vi "PS_Pressure_Cal.vi"(11 "P":dbl=1.0) -> (0 "error out":errorcluster, 3 "Pn":dbl)   [LabVIEW 2011]
uses:
  PS_Global.vi
panel:
  # "torr"
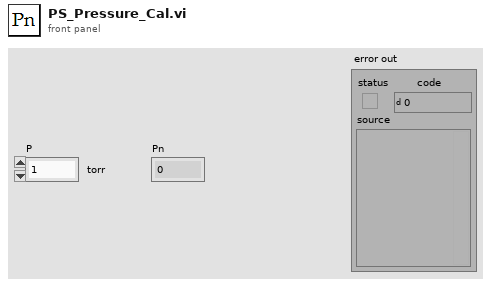
[diagram p1: front panel]
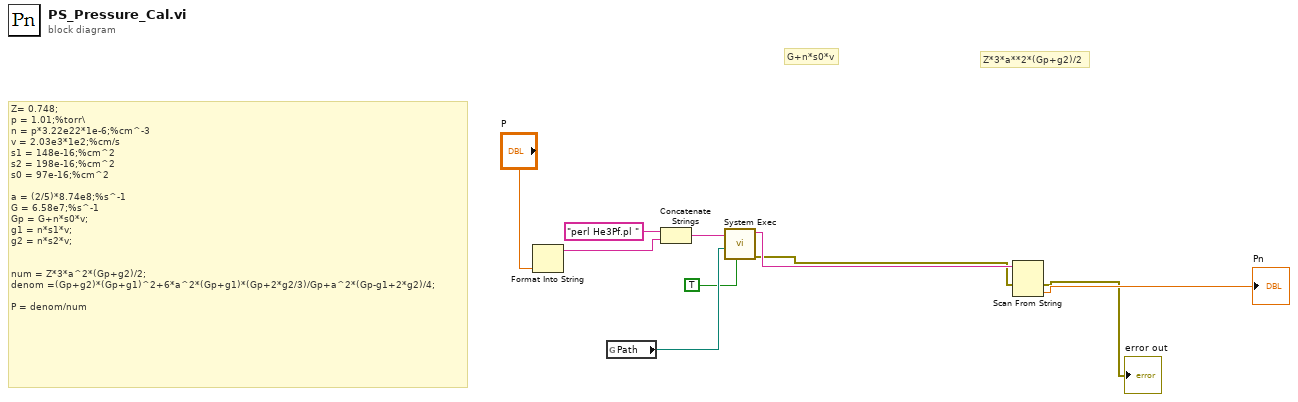
[diagram p0: block diagram]
diagram:
  # "G+n*s0*v"
  # "Z*3*a**2*(Gp+g2)/2"
  # "Z= 0.748;\np = 1.01;%torr\\\nn = p*3.22e22*1e-6;%cm^-3\nv = 2.03e3*1e2;%cm/s\ns1 = 148e-16;%cm^2\ns2 = 198e-16;%cm^2\ns0 = 97e-16;%cm^2\n\na = (2/5)*8.74e8;%s^-1\nG = 6.58e7;%s^-1\nGp = G+n*s0*v;\ng1 = n*s1*v;\ng2 = n*s2*v;\n\n\nnum = Z*3*a^2*(Gp+g2)/2;\ndenom =(Gp+g2)*(Gp+g1)^2+6*a^2*(Gp+g1)*(Gp+2*g2/3)/Gp+a^2*(Gp-g1+2*g2)/4;\n\nP = denom/num"
  n1 = Format Into String("P") -> (resulting string=w7:string)  [unwired: 3 in, 1 out]
  n2 = global read "PS_Global.vi" "Path"() -> (w4:path)
  n3 = Concatenate Strings("perl He3Pf.pl " ("string"), w7) -> (w10:string)
  n4 = call <vilib>:"System Exec.vi"("run minimized? (F)"=TRUE, "working directory"=w4, "command line"=w10) -> ("error out"=w3:errorcluster, "standard output"=w5:string)  [unwired: 5 in, 2 out]
  n5 = Scan From String(input string=w5, error in=w3) -> (error out=→"error out":errorcluster, output 1=→"Pn":dbl)  [unwired: 3 in, 2 out]
